vi "SetProcessRunStatus.vi"(8 "error in":errorcluster, 10 "ProcessRunStatus":T1=enum."NOT_COMPLETED", 11 "ProcessRun in":refnum<class "ProcessRun.lvclass">) -> (0 "error out":errorcluster, 3 "ProcessRun out":refnum<class "ProcessRun.lvclass">)   [LabVIEW 2021, in "ProligentXMLGenerator.lvlib" / "ProcessRun.lvclass"]
doc: "Defines the last known status of the operation run.\n\nPASS: The execution completed successfully.\nFAIL: The execution completed and failures were detected.\nNOT_COMPLETED: The execution is not completed. It is still in progress. In that situation, the end time of the execution must be ommited.\nABORTED: The execution was aborted."
uses:
  ProcessRun.lvclass
  ProcessRun.lvclass/ProcessRun.ctl
  Base/ExecutionStatus/Value.ctl
  Base/ExecutionStatus/ExecutionStatus.lvclass
  Base/DateTime/DateTime.lvclass
  Base/Attribute/Attribute.lvclass
  C:/Projects/proligent-xml-generator-labview/src/ProligentXMLGenerator/Base/Attribute/Attribute.lvclass
  C:/Projects/proligent-xml-generator-labview/src/ProligentXMLGenerator/Base/DateTime/DateTime.lvclass
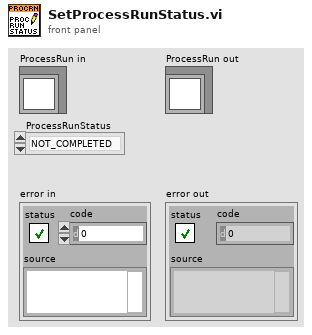
[diagram p1: front panel]
types:
  T1 = typedef "ProligentXMLGenerator.lvlib/ExecutionStatus.lvclass/Value.ctl" = enum16{"PASS", "FAIL", "NOT_COMPLETED", "ABORTED"}
  T2 = typedef "ProligentXMLGenerator.lvlib/ProcessRun.lvclass/Data.ctl" = cluster{"Name":string, "OperationRuns":refnum<class "OperationRun.lvclass">[], "OperationCycles":refnum<class "OperationCycle.lvclass">[], "FailureReferences":refnum<class "FailureReference.lvclass">[], "CustomData":refnum<class "CustomData.lvclass">, "ProcessRunId":refnum<class "Guid.lvclass">, "ProcessFullName":refnum<class "ProcessFullName.lvclass">, "ProcessVersion":refnum<class "NonEmptyString_64.lvclass">, "ProductUnitIdentifier":refnum<class "NonEmptyString_50.lvclass">, "ProductFullName":refnum<class "FullName.lvclass">, "ProcessRunStatus":refnum<class "ExecutionStatus.lvclass">, "ProcessRunStartTime":refnum<class "DateTime.lvclass">, "ProcessRunEndTime":refnum<class "DateTime.lvclass">, "ProcessMode":refnum<class "NonEmptyString_64.lvclass">, "TimeZoneInfoId":string}
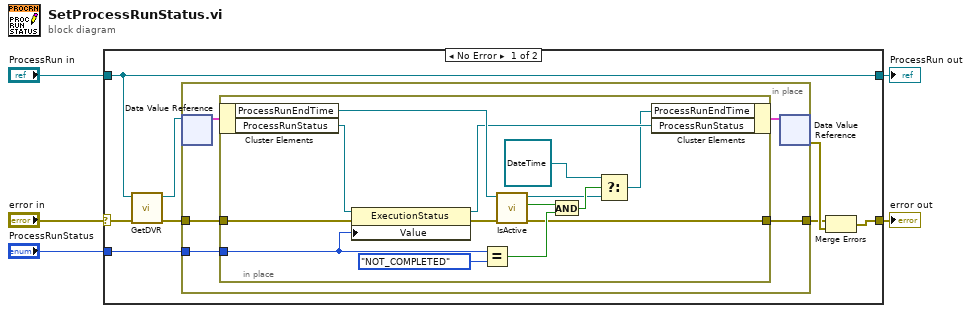
[diagram p0: block diagram]
diagram:
  n1 = case shown="No Error" "error in" {
    selector: "error in" -> [w11 w33]
    tunnel: "ProcessRun in" -> [w6 w34]
    tunnel: [w8 w33] -> w3
    tunnel: "ProcessRunStatus" -> [w7 _]
    tunnel: [w6 w34] -> w1
    frame No Error {
      n2 = call "GetDVR.vi"("error in"=w11, "ProcessRun"=w6) -> ("error out"=w10:errorcluster, "DVRReference"=w12:refnum<data-value>)  [unwired: 8 in]
      n3 = in-place "In Place Element Structure" {
        in-place-border: w10 -> [w18]
        in-place-border: [w16] -> w9
        in-place-border: w7 -> [w17]
        n4 = in-place-dvr #1(w12) -> (w15:T2)  [unwired: 1 out]
        n5 = in-place "In Place Element Structure" {
          in-place-border: w18 -> [w32]
          in-place-border: w17 -> [w31]
          in-place-border: [w26] -> w16
          n6 = in-place-cluster #2(w15) -> ("ProcessRunEndTime"=w24:refnum<class "DateTime.lvclass">, "ProcessRunStatus"=w25:refnum<class "ExecutionStatus.lvclass">)
          n7 = property on="Property Node" class="ExecutionStatus"(reference=w25, error in=w32, "Value"=w31) -> (reference out=w23:refnum<class "ExecutionStatus.lvclass">, error out=w29:errorcluster)
          n8 = Equal?(x=w31, y=Value."NOT_COMPLETED") -> (x = y?=w27:bool)
          n9 = call "IsActive.vi"("error in"=w29, "Attribute in"=w24) -> ("error out"=w26:errorcluster, "IsActive"=w28:bool, "Attribute in"=w21:refnum<class "DateTime.lvclass">)  [unwired: 7 in]
          n10 = And(x=w28, y=w27) -> (x .and. y?=w22:bool)
          n11 = Select(t=refnum<class "DateTime.lvclass"> refnum ("ProcessRunEndTime"), s=w22, f=w21) -> (s? t:f=w19:refnum<class "DateTime.lvclass">)
          n12 = in-place-cluster #2("ProcessRunEndTime"=w19, "ProcessRunStatus"=w23) -> (w14:T2)
        }
        n13 = in-place-dvr #1(w14) -> (w13:errorcluster)  [unwired: 1 out]
      }
      n14 = Merge Errors(w9, w13) -> (w8:errorcluster)
    }
    frame Error {
    }
  }
  "error out" <- w3
  "ProcessRun out" <- w1
